vi "fault notifications.vi"(0 "Dismiss Notification":bool, 5 "Hardware Fault":bool, 7 "Temperature Fault":bool, 9 "Battery Voltage Fault":bool, 11 "Current Faults":bool[](array[boolean])=[FALSE, FALSE, FALSE, FALSE, FALSE, FALSE, FALSE, FALSE, FALSE, FALSE, FALSE, FALSE, FALSE, FALSE, FALSE, FALSE], 12 "Compressor Fault":bool, 13 "All Solenoid Faults":bool[](array[boolean])=[FALSE, FALSE, FALSE, FALSE, FALSE, FALSE, FALSE, FALSE], 14 "roboRIO Faults":T1) -> (4 "Notification":string, 10 "Blinking?":bool, 15 "Visible?":bool)   [LabVIEW 2014]
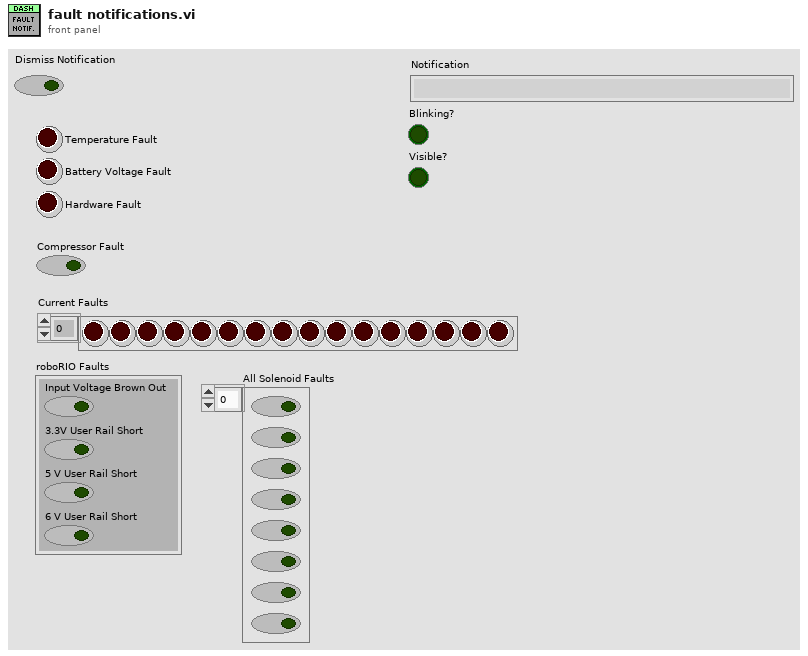
[diagram p1: front panel]
types:
  T1 = cluster{"Input Voltage Brown Out":bool, "3.3V User Rail Short":bool, "5 V User Rail Short":bool, "6 V User Rail Short":bool}
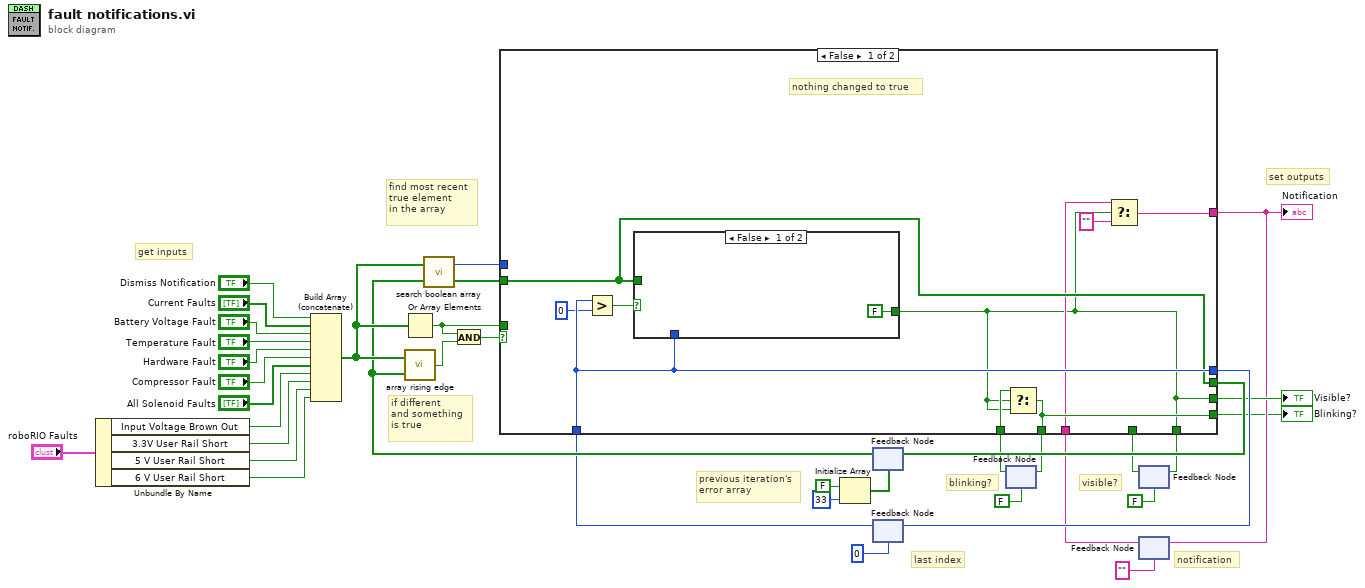
[diagram p0: block diagram]
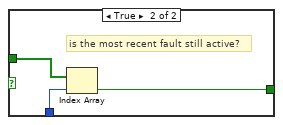
[diagram p2: hidden frame]
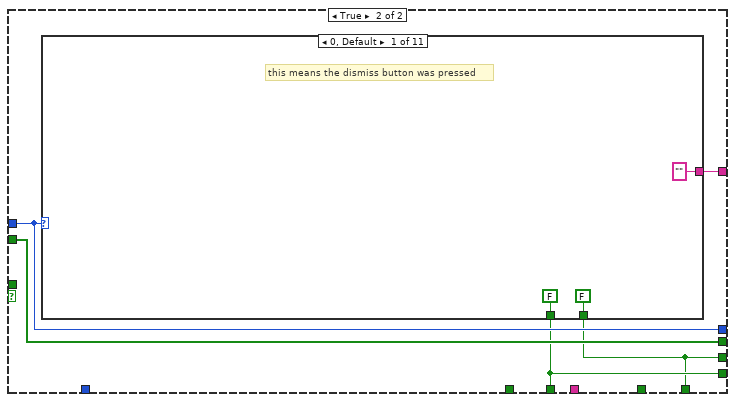
[diagram p3: hidden frame]
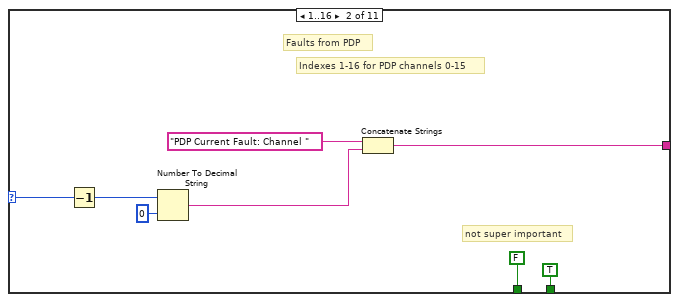
[diagram p4: hidden frame]
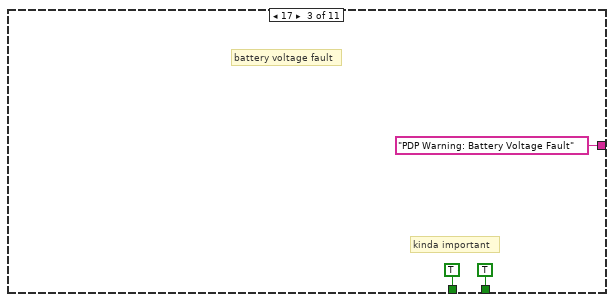
[diagram p5: hidden frame]
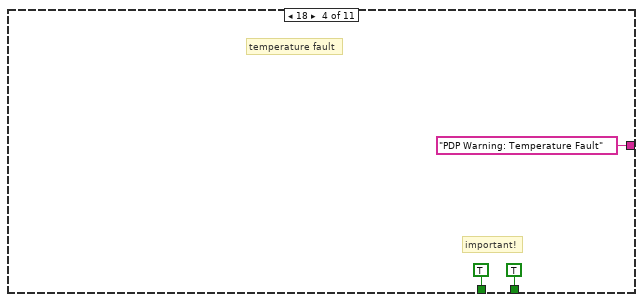
[diagram p6: hidden frame]
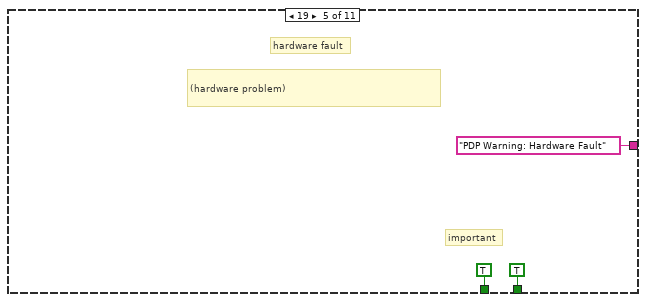
[diagram p7: hidden frame]
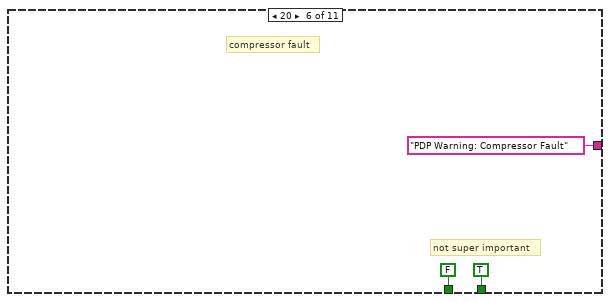
[diagram p8: hidden frame]
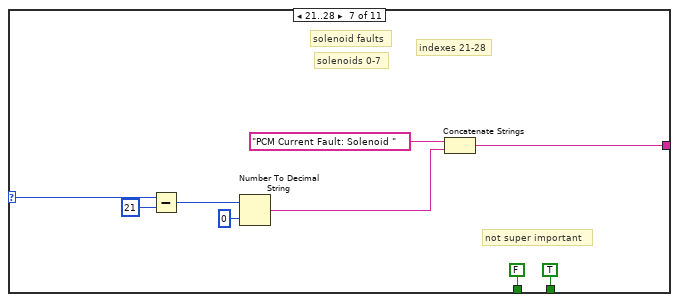
[diagram p9: hidden frame]
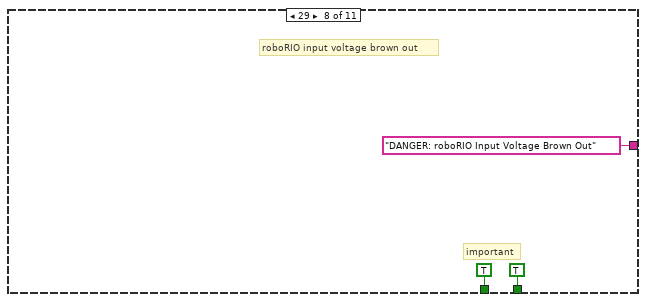
[diagram p10: hidden frame]
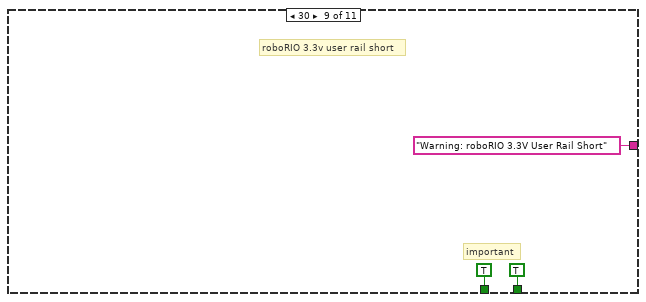
[diagram p11: hidden frame]
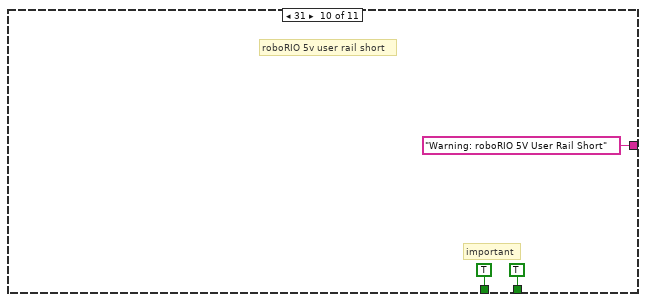
[diagram p12: hidden frame]
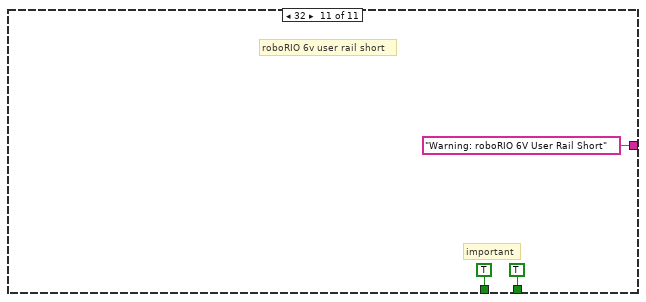
[diagram p13: hidden frame]
diagram:
  # "set outputs"
  # "get inputs"
  # "if different\nand something\nis true"
  # "find most recent\ntrue element\nin the array"
  # "notification"
  # "blinking?"
  # "previous iteration's\nerror array"
  # "last index"
  # "visible?"
  n1 = Unbundle By Name("roboRIO Faults") -> ("Input Voltage Brown Out"=w24:bool, "3.3V User Rail Short"=w23:bool, "5 V User Rail Short"=w22:bool, "6 V User Rail Short"=w21:bool)
  n2 = Build Array (concatenate)("Dismiss Notification", "Current Faults", "Battery Voltage Fault", "Temperature Fault", "Hardware Fault", "Compressor Fault", "All Solenoid Faults", w24, w23, w22, w21) -> (w4:bool[])
  n3 = Or Array Elements(Boolean array=w4) -> (logical OR=w1:bool)
  n4 = Initialize Array(FALSE ("Hardware Fault"), 33 ("dimension size")) -> (w8:bool[])
  n5 = feedback #1(w8) -> (w3:bool[])
  n6 = call "array rising edge.vi"("Previous Array"=w3, "Current Array"=w4) -> ("Update Display"=w5:bool)
  n7 = call "search boolean array.vi"("Previous Array"=w3, "Array In"=w4) -> ("Array Out"=w11:bool[], "Index"=w31:i32)
  n8 = And(x=w1, y=w5) -> (x .and. y?=w7:bool)
  n9 = feedback #2(0 ("Button Pressed")) -> (w2:i32)
  n10 = feedback #3(FALSE) -> (w15:bool)
  n11 = feedback #4(FALSE) -> (w18:bool)
  n12 = feedback #5("") -> (w13:string)
  n13 = case shown="False" w7 {
    tunnel: [w42 w55] -> w32
    tunnel: w31 -> [_ w54]
    tunnel: [w45 w54] -> w30
    tunnel: w2 -> [w45 _]
    tunnel: [w39 w52] -> w28
    tunnel: [w39 w52] -> w19
    tunnel: w18 -> [_ _]
    tunnel: [w46 w53] -> w16
    tunnel: w15 -> [w47 _]
    tunnel: [w41 w56] -> w14
    tunnel: w13 -> [w40 _]
    tunnel: w11 -> [w42 w55]
    tunnel: [w46 w53] -> w6
    tunnel: w1 -> [_ _]
    frame False {
      # "nothing changed to true"
      n14 = Greater?(x=w45, y=0) -> (0:w43:bool)
      n15 = case shown="False" w43 {
        tunnel: w42 -> [_ w51]
        tunnel: w45 -> [_ w50]
        tunnel: [FALSE ("Boolean") w49] -> w39
        frame False {
        }
        frame True {
          # "is the most recent fault still active?"
          n16 = Index Array(array=w51, index=w50) -> (element=w49:bool)
        }
      }
      n17 = Select(t=w47, s=w39, f=w39) -> (s? t:f=w46:bool)
      n18 = Select(t=w40, s=w39, f="") -> (s? t:f=w41:string)
    }
    frame True {
      n19 = case shown="0, Default" w54 {
        selector: w54 -> [_ w62 _ _ _ _ w84 _ _ _ _]
        tunnel: [FALSE FALSE TRUE TRUE TRUE FALSE FALSE TRUE TRUE TRUE TRUE] -> w53
        tunnel: ["" w64 "PDP Warning: Battery Voltage Fault" "PDP Warning: Temperature Fault" "PDP Warning: Hardware Fault" "PDP Warning: Compressor Fault" w82 "DANGER: roboRIO Input Voltage Brown Out" "Warning: roboRIO 3.3V User Rail Short" "Warning: roboRIO 5V User Rail Short" "Warning: roboRIO 6V User Rail Short"] -> w56
        tunnel: [FALSE TRUE TRUE TRUE TRUE TRUE TRUE TRUE TRUE TRUE TRUE] -> w52
        frame 0, Default {
          # "this means the dismiss button was pressed"
        }
        frame 1..16 {
          # "not super important"
          # "Indexes 1-16 for PDP channels 0-15"
          # "Faults from PDP"
          n20 = Decrement(x=w62) -> (x-1=w63:i32)
          n21 = Number To Decimal String(number=w63, width (-)=i16 0) -> (decimal integer string=w65:string)
          n22 = Concatenate Strings("PDP Current Fault: Channel ", w65) -> (w64:string)
        }
        frame 17 {
          # "kinda important"
          # "battery voltage fault"
        }
        frame 18 {
          # "important!"
          # "temperature fault"
        }
        frame 19 {
          # "important"
          # "(hardware problem)"
          # "hardware fault"
        }
        frame 20 {
          # "not super important"
          # "compressor fault"
        }
        frame 21..28 {
          # "not super important"
          # "indexes 21-28"
          # "solenoids 0-7"
          # "solenoid faults"
          n23 = Subtract(x=w84, y=21) -> (x-y=w85:i32)
          n24 = Number To Decimal String(number=w85, width (-)=i16 0) -> (decimal integer string=w86:string)
          n25 = Concatenate Strings("PCM Current Fault: Solenoid ", w86) -> (w82:string)
        }
        frame 29 {
          # "important"
          # "roboRIO input voltage brown out"
        }
        frame 30 {
          # "important"
          # "roboRIO 3.3v user rail short"
        }
        frame 31 {
          # "important"
          # "roboRIO 5v user rail short"
        }
        frame 32 {
          # "important"
          # "roboRIO 6v user rail short"
        }
      }
    }
  }
  "Notification" <- w14
  "Visible?" <- w28
  "Blinking?" <- w6
  n26 = feedback-in #1(w32) -> ()
  n27 = feedback-in #2(w30) -> ()
  n28 = feedback-in #3(w16) -> ()
  n29 = feedback-in #4(w19) -> ()
  n30 = feedback-in #5(w14) -> ()
